vi "Read Graph-Chart Axis Labels.vi"(8 "error in":errorcluster, 11 "Graph / Chart Reference in":refnum<vi>) -> (0 "error out":errorcluster, 1 "X Axis":string, 2 "Interpret As Unicode (X)":bool, 3 "Graph / Chart Reference out":refnum<vi>, 4 "Interpret As Unicode (Y)":bool, 6 "Y Axis":string)   [LabVIEW 2020, in "G-Unicode.lvlib"]
uses:
  G-Unicode.lvlib
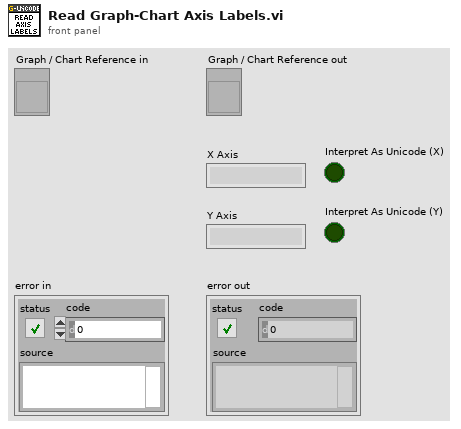
[diagram p1: front panel]
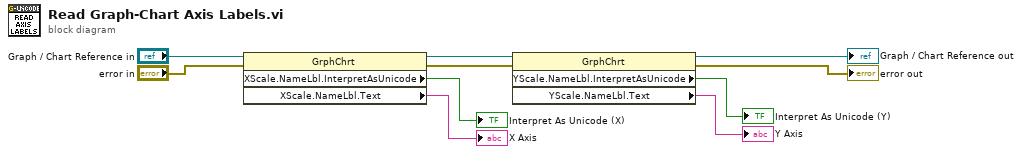
[diagram p0: block diagram]
diagram:
  n1 = property class="GrphChrt"(reference="Graph / Chart Reference in", error in="error in") -> (reference out=w8:refnum<vi>, error out=w6:errorcluster, "XScale.NameLbl.InterpretAsUnicode"=→"Interpret As Unicode (X)":bool, "XScale.NameLbl.Text"=→"X Axis":string)
  n2 = property class="GrphChrt"(reference=w8, error in=w6) -> (reference out=→"Graph / Chart Reference out":refnum<vi>, error out=→"error out":errorcluster, "YScale.NameLbl.InterpretAsUnicode"=→"Interpret As Unicode (Y)":bool, "YScale.NameLbl.Text"=→"Y Axis":string)
